vi "Main.vi"(8 "error in":errorcluster, 11 "TopUI in":refnum<class "TopUI.lvclass">) -> (0 "error out":errorcluster, 3 "TopUI out":refnum<class "TopUI.lvclass">)   [LabVIEW 2024, in "TopUI.lvclass"]
doc: "The <b>Queued Message Handler</b> of the Worker that owns this VI."
uses:
  TopUI.lvclass
  C:/Program Files (x86)/National Instruments/LabVIEW 2024/vi.lib/addons/_Workers/Library/Classes/Worker/Worker.lvclass
  TopUI.lvclass/TopUI.ctl
  Initialization Data.ctl
  Response Cases.ctl
  rql_NewAPIMHLCreate.ctl
  rql_UpdatePanelDisplay.ctl
  rql_ReadMeterValue.ctl
  rql_GetValueAvg.ctl
  <vilib>/addons/_Workers/Library/Classes/Message Queue/Message Queue.lvclass
  ooxxMeter/ooxxMeter.lvclass
  C:/Program Files (x86)/National Instruments/LabVIEW 2024/vi.lib/addons/_Workers/Library/Classes/Workers Object/Workers Object.lvclass
  C:/Users/chrismadlax/Desktop/LVSampleCode/Wokers50Demo/Workers/TopUI/TopUI.lvclass
panel:
  out "ValueAvg":dbl
  in  "GetValueAvg":bool
  out "MeterValue":dbl
  in  "ReadMeter":bool
  in  "Increment":bool
  out "Counter":dbl
  # "Public Request with respones"
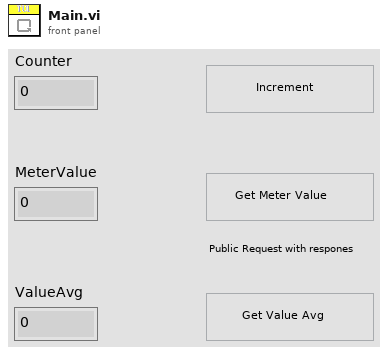
[diagram p1: front panel]
types:
  T1 = typedef "TopUI.lvclass/Initialization Data.ctl" = cluster{"Response Cases":T2}
  T2 = typedef "TopUI.lvclass/Response Cases.ctl" = cluster{"Placeholder - Can be deleted":string}
  T3 = typedef "TopUI.lvclass/rql_NewAPIMHLCreate.ctl" = cluster{"String":string}
  T4 = typedef "TopUI.lvclass/rql_UpdatePanelDisplay.ctl" = cluster{"String":string}
  T5 = typedef "TopUI.lvclass/rql_ReadMeterValue.ctl" = cluster{"String":string}
  T6 = typedef "TopUI.lvclass/rql_GetValueAvg.ctl" = cluster{"String":string}
  T7 = typedef "ooxxMeter.lvclass/rwr_ReadMeterValueNow Reply.ctl" = cluster{"String":string, "MeterValue":dbl}
  T8 = typedef "ooxxMeter.lvclass/rsp_ReturnValueAvg.ctl" = cluster{"String":string, "ValueAvg":dbl}
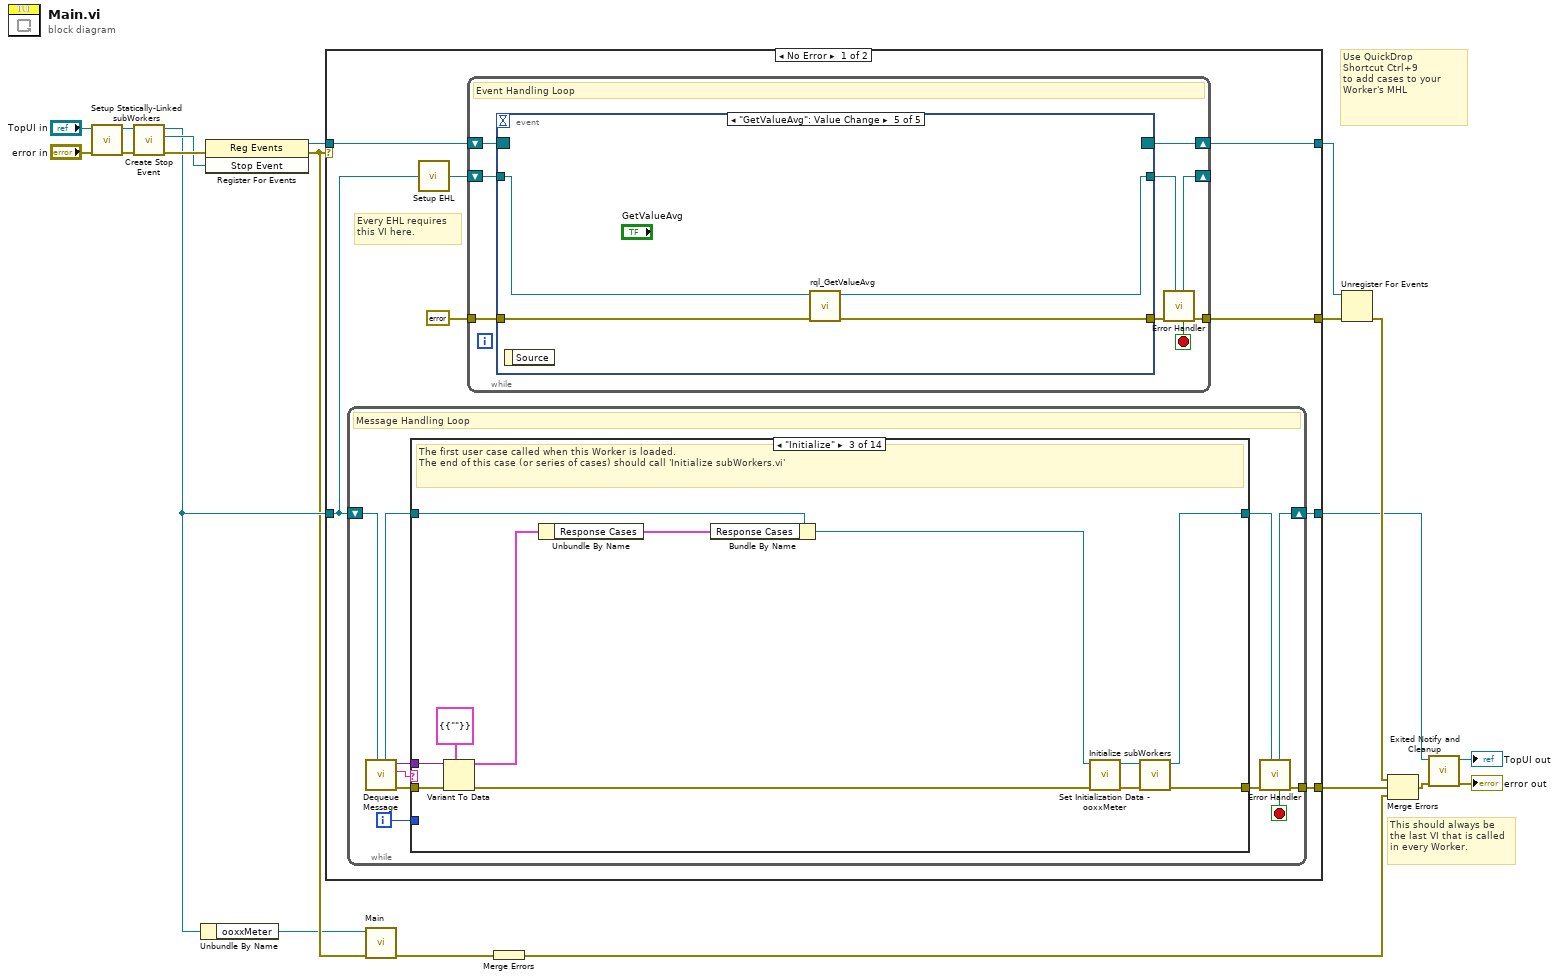
[diagram p0: block diagram]
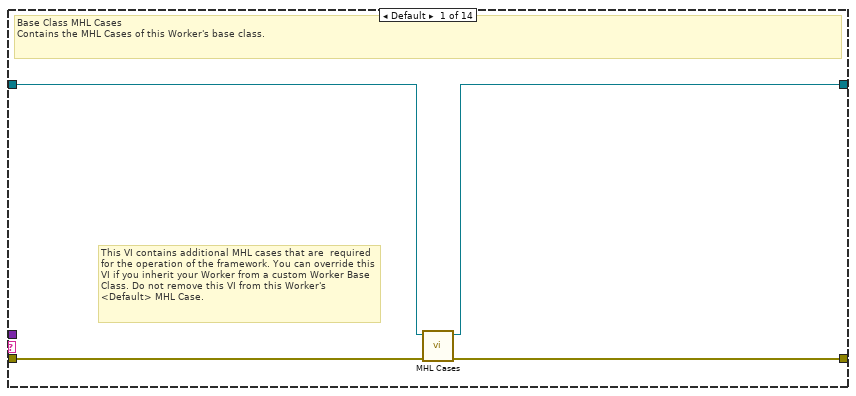
[diagram p2: hidden frame]
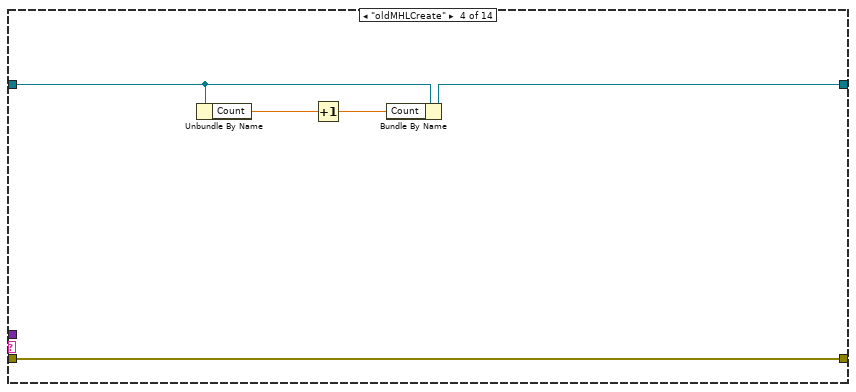
[diagram p4: hidden frame]
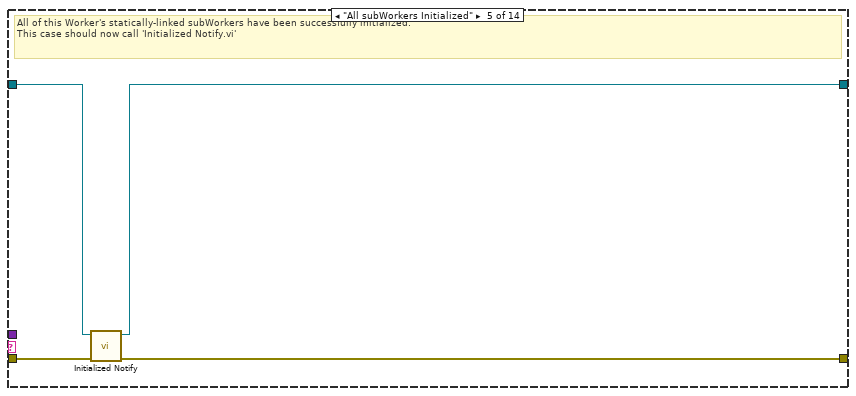
[diagram p5: hidden frame]
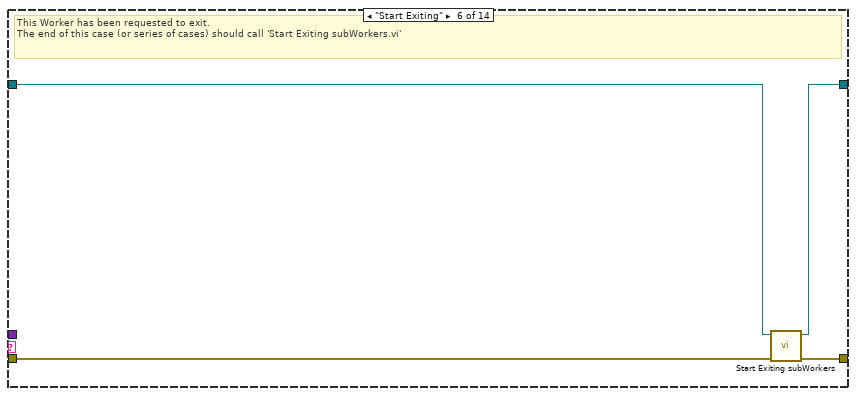
[diagram p6: hidden frame]
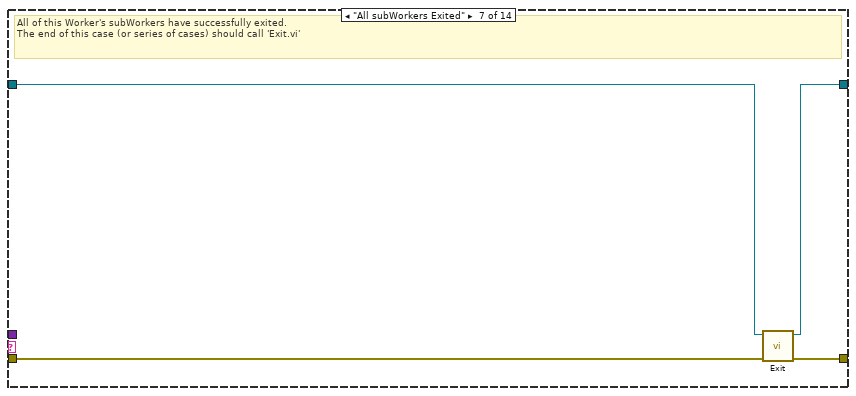
[diagram p7: hidden frame]
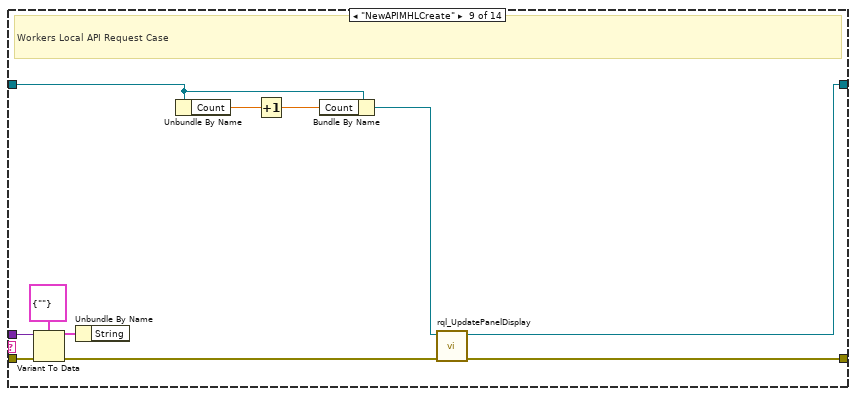
[diagram p9: hidden frame]
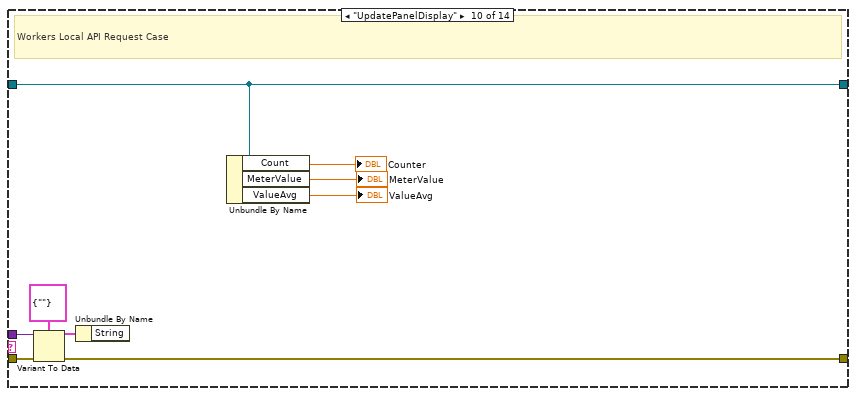
[diagram p10: hidden frame]
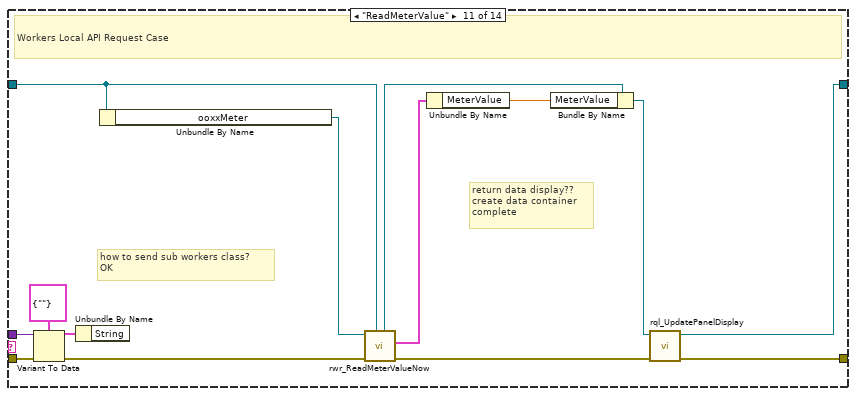
[diagram p11: hidden frame]
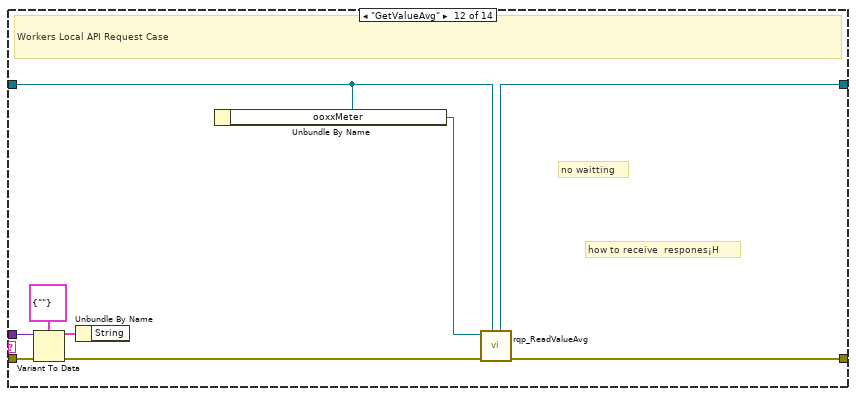
[diagram p12: hidden frame]
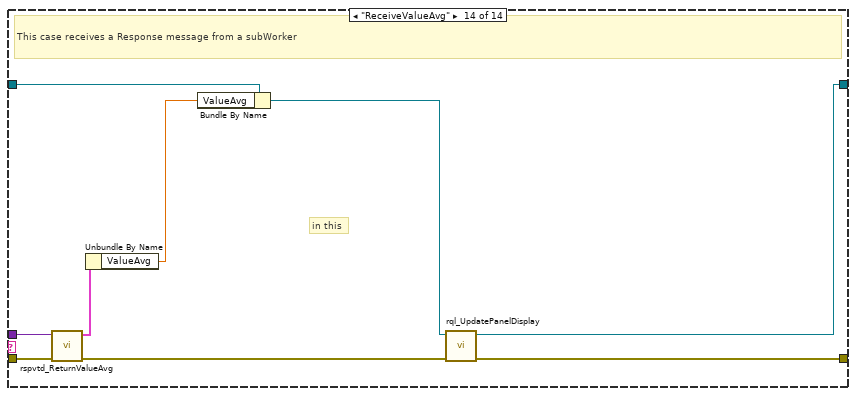
[diagram p14: hidden frame]
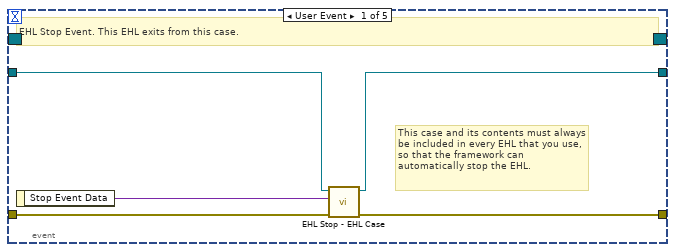
[diagram p15: hidden frame]
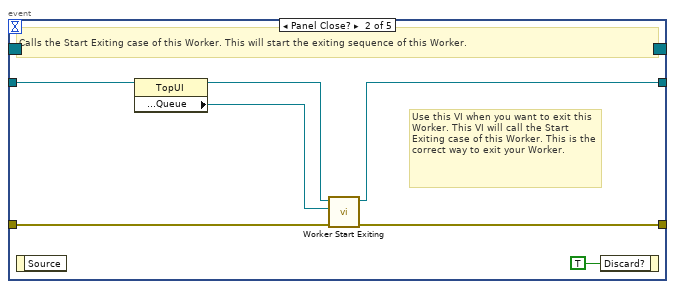
[diagram p16: hidden frame]
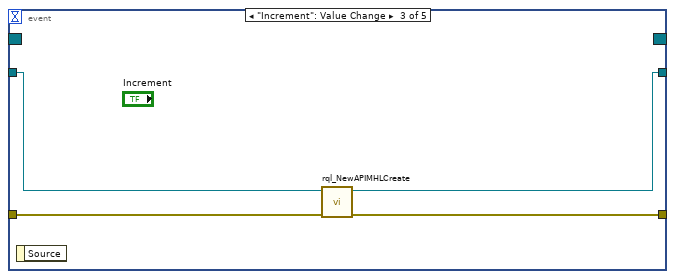
[diagram p17: hidden frame]
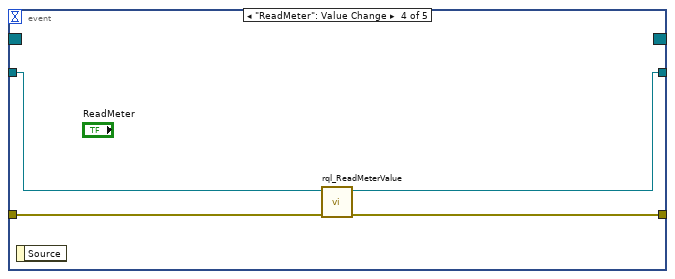
[diagram p18: hidden frame]
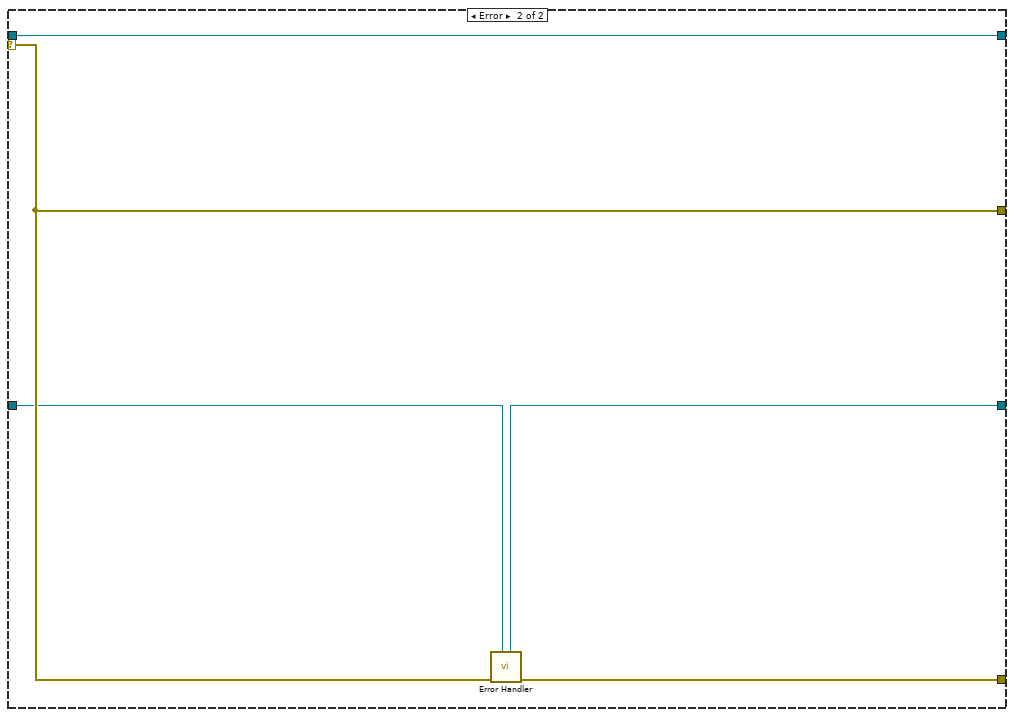
[diagram p19: hidden frame]
diagram:
  # "Use QuickDrop\nShortcut Ctrl+9\nto add cases to your\nWorker's MHL"
  # "This should always be the last VI that is called in every Worker."
  n1 = call "Setup Statically-Linked subWorkers.vi"("error in"="error in", "TopUI in"="TopUI in") -> ("error out"=w6:errorcluster, "TopUI out"=w4:refnum<class "TopUI.lvclass">)  [unwired: 8 in]
  n2 = call-dynamic "Create Stop Event.vi"("error in"=w6, "Worker"=w4) -> ("error out"=w15:errorcluster, "Stop Event"=w12:refnum<user-event>, "Worker out"=w9:refnum<class "TopUI.lvclass">)  [unwired: 7 in]
  n3 = Unbundle By Name(w9) -> ("ooxxMeter"=w1:refnum<class "ooxxMeter.lvclass">)
  n4 = register-events(error in=w15, w12) -> (reference out=w14:refnum<event-registration>, error out=w7:errorcluster)  [unwired: 1 in]
  n5 = case shown="No Error" w7 {
    tunnel: w9 -> [w23 w165]
    tunnel: [w21 w166] -> w13
    tunnel: w14 -> [w28 w167]
    tunnel: [w25 w168] -> w19
    tunnel: [w27 w167] -> w18
    tunnel: [w22 w164] -> w16
    selector: w7 -> [_ w168]
    frame No Error {
      # "Every EHL requires\nthis VI here."
      n6 = while {
        shift-right: [w37] -> w22
        shift-left: w23 -> [w39]
        tunnel: [w38] -> w21
        i -> [w30]
        stop <- w31 stop-if-true
        # "Message Handling Loop"
        n7 = call-dynamic "Dequeue Message.vi"("Worker"=w39) -> ("error out"=w36:errorcluster, "Case out"=w32:string, "Data out"=w29:variant, "Worker out"=w34:refnum<class "TopUI.lvclass">)  [unwired: 6 in, 1 out]
        n8 = case "Worker MHL Case Structure (DO NOT CHANGE LABEL NAME)" shown="\"Initialize\"" w32 {
          tunnel: w36 -> [w43 w44 w55 w62 w64 w67 w74 w76 w87 w96 w110 w119 w121 w130]
          tunnel: [w42 w44 w57 w62 w63 w70 w73 w76 w79 w95 w99 w114 w121 w124] -> w35
          tunnel: w34 -> [w41 w45 w54 w60 w66 w68 w72 w75 w82 w91 w103 w112 w120 w129]
          tunnel: [w40 w45 w56 w61 w65 w69 w71 w75 w77 w91 w97 w113 w120 w122] -> w33
          tunnel: w30 -> [_ _ _ _ _ _ _ _ _ _ _ _ _ _]
          tunnel: w29 -> [_ _ w52 _ _ _ _ _ w84 w93 w107 w116 _ w127]
          frame Default {
            # "This VI contains additional MHL cases that are  required for the operation of the framework. You can override this VI if you inherit your Worker from a custom Worker Base Class. Do not remove this VI from this Worker's <Default> MHL Case."
            # "Base Class MHL Cases\nContains the MHL Cases of this Worker's base class."
            n9 = call-dynamic "MHL Cases.vi"("error in"=w43, "Worker in"=w41) -> ("error out"=w42:errorcluster, "Worker out"=w40:refnum<class "TopUI.lvclass">)  [unwired: 8 in]
          }
          frame "------------ FRAMEWORK CASES -----------" {
            # "Start of Workers Framework Cases"
          }
          frame "Initialize" {
            # "The first user case called when this Worker is loaded.\nThe end of this case (or series of cases) should call 'Initialize subWorkers.vi'"
            n10 = Variant To Data(error in=w55, type=T1 {"Response Cases"={"Placeholder - Can be deleted"=""}} ("Initialization Data"), Variant=w52) -> (data=w51:T1, error out=w53:errorcluster)
            n11 = Unbundle By Name(w51) -> ("Response Cases"=w50:T2)
            n12 = Bundle By Name(cluster=w54, "Response Cases"=w50) -> (w46:refnum<class "TopUI.lvclass">)
            n13 = call "Set Initialization Data - ooxxMeter.vi"("error in"=w53, "TopUI in"=w46) -> ("error out"=w48:errorcluster, "TopUI out"=w47:refnum<class "TopUI.lvclass">)  [unwired: 8 in]
            n14 = call-dynamic "Initialize subWorkers.vi"("error in"=w48, "Worker"=w47) -> ("error out"=w57:errorcluster, "dup Worker out"=w56:refnum<class "TopUI.lvclass">)  [unwired: 8 in]
          }
          frame "oldMHLCreate" {
            n15 = Unbundle By Name(w60) -> ("Count"=w59:dbl)
            n16 = Increment(x=w59) -> (x+1=w58:dbl)
            n17 = Bundle By Name(cluster=w60, "Count"=w58) -> (w61:refnum<class "TopUI.lvclass">)
          }
          frame "All subWorkers Initialized" {
            # "All of this Worker's statically-linked subWorkers have been successfully initialized.\nThis case should now call 'Initialized Notify.vi'"
            n18 = call-dynamic "Initialized Notify.vi"("error in"=w64, "Worker"=w66) -> ("error out"=w63:errorcluster, "dup Worker out"=w65:refnum<class "TopUI.lvclass">)  [unwired: 8 in]
          }
          frame "Start Exiting" {
            # "This Worker has been requested to exit. \nThe end of this case (or series of cases) should call 'Start Exiting subWorkers.vi'"
            n19 = call-dynamic "Start Exiting subWorkers.vi"("error_in"=w67, "Worker"=w68) -> ("error out"=w70:errorcluster, "dup Worker out"=w69:refnum<class "TopUI.lvclass">)  [unwired: 8 in]
          }
          frame "All subWorkers Exited" {
            # "All of this Worker's subWorkers have successfully exited. \nThe end of this case (or series of cases) should call 'Exit.vi'"
            n20 = call-dynamic "Exit.vi"("error_in"=w74, "Worker"=w72) -> ("error out"=w73:errorcluster, "dup Worker out"=w71:refnum<class "TopUI.lvclass">)  [unwired: 8 in]
          }
          frame "------------- LOCAL API CASES -------------" {
            # "Start of Workers Local API Cases"
          }
          frame "NewAPIMHLCreate" {
            # "Workers Local API Request Case"
            n21 = Variant To Data(error in=w87, type=T3 {"String"=""} ("Data"), Variant=w84) -> (data=w83:T3, error out=w86:errorcluster)
            n22 = Unbundle By Name(w83) -> ()  [unwired: 1 out]
            n23 = Unbundle By Name(w82) -> ("Count"=w81:dbl)
            n24 = Increment(x=w81) -> (x+1=w80:dbl)
            n25 = Bundle By Name(cluster=w82, "Count"=w80) -> (w78:refnum<class "TopUI.lvclass">)
            n26 = call "rql_UpdatePanelDisplay.vi"("error in"=w86, "TopUI in"=w78) -> ("error out"=w79:errorcluster, "dup TopUI out"=w77:refnum<class "TopUI.lvclass">)  [unwired: 8 in]
          }
          frame "UpdatePanelDisplay" {
            # "Workers Local API Request Case"
            n27 = Variant To Data(error in=w96, type=T4 {"String"=""} ("Data"), Variant=w93) -> (data=w92:T4, error out=w95:errorcluster)
            n28 = Unbundle By Name(w92) -> ()  [unwired: 1 out]
            n29 = Unbundle By Name(w91) -> ("Count"=→"Counter":dbl, "MeterValue"=→"MeterValue":dbl, "ValueAvg"=→"ValueAvg":dbl)
          }
          frame "ReadMeterValue" {
            # "return data display??\ncreate data container\ncomplete"
            # "how to send sub workers class?\nOK"
            # "Workers Local API Request Case"
            n30 = Variant To Data(error in=w110, type=T5 {"String"=""} ("Data"), Variant=w107) -> (data=w106:T5, error out=w109:errorcluster)
            n31 = Unbundle By Name(w106) -> ()  [unwired: 1 out]
            n32 = Unbundle By Name(w103) -> ("ooxxMeter"=w102:refnum<class "ooxxMeter.lvclass">)
            n33 = call "rwr_ReadMeterValueNow.vi"("Caller in"=w103, "error in"=w109, "ooxxMeter in"=w102) -> ("error out"=w105:errorcluster, "Reply Data out"=w101:T7, "dup Caller out"=w104:refnum<class "TopUI.lvclass">)  [unwired: 5 in, 1 out]
            n34 = Unbundle By Name(w101) -> ("MeterValue"=w100:dbl)
            n35 = Bundle By Name(cluster=w104, "MeterValue"=w100) -> (w98:refnum<class "TopUI.lvclass">)
            n36 = call "rql_UpdatePanelDisplay.vi"("error in"=w105, "TopUI in"=w98) -> ("error out"=w99:errorcluster, "dup TopUI out"=w97:refnum<class "TopUI.lvclass">)  [unwired: 8 in]
          }
          frame "GetValueAvg" {
            # "how to receive  respones¡H"
            # "no waitting"
            # "Workers Local API Request Case"
            n37 = Variant To Data(error in=w119, type=T6 {"String"=""} ("Data"), Variant=w116) -> (data=w115:T6, error out=w118:errorcluster)
            n38 = Unbundle By Name(w115) -> ()  [unwired: 1 out]
            n39 = Unbundle By Name(w112) -> ("ooxxMeter"=w111:refnum<class "ooxxMeter.lvclass">)
            n40 = call "rqp_ReadValueAvg.vi"("Caller in"=w112, "error in"=w118, "ooxxMeter in"=w111) -> ("error out"=w114:errorcluster, "dup Caller out"=w113:refnum<class "TopUI.lvclass">)  [unwired: 6 in, 1 out]
          }
          frame "------------- RESPONSE CASES --------------" {
            # "Start of Workers Response Cases"
          }
          frame "ReceiveValueAvg" {
            # "in this"
            # "This case receives a Response message from a subWorker"
            n41 = call "rspvtd_ReturnValueAvg.vi"("error in"=w130, "Data in"=w127) -> ("error out"=w128:errorcluster, "Data out"=w126:T8)  [unwired: 8 in]
            n42 = Unbundle By Name(w126) -> ("ValueAvg"=w125:dbl)
            n43 = Bundle By Name(cluster=w129, "ValueAvg"=w125) -> (w123:refnum<class "TopUI.lvclass">)
            n44 = call "rql_UpdatePanelDisplay.vi"("error in"=w128, "TopUI in"=w123) -> ("error out"=w124:errorcluster, "dup TopUI out"=w122:refnum<class "TopUI.lvclass">)  [unwired: 8 in]
          }
        }
        n45 = call-dynamic "Error Handler.vi"("Worker"=w33, "error_in"=w35) -> ("error out"=w38:errorcluster, "Stop Loop"=w31:bool, "Worker out"=w37:refnum<class "TopUI.lvclass">)  [unwired: 7 in]
      }
      n46 = call-dynamic "Setup EHL.vi"("Worker"=w23) -> ("Worker out"=w24:refnum<class "TopUI.lvclass">)  [unwired: 14 in]
      n47 = while "Event Handling Loop" {
        shift-right: [w139] -> w27
        shift-left: w28 -> [w138]
        tunnel: [w134] -> w25
        tunnel: errorcluster {"status"=FALSE, "code"=0, "source"=""} ("error constant") -> [w136]
        shift-right: [w132] -> _
        shift-left: w24 -> [w137]
        stop <- w131 stop-if-true
        # "Event Handling Loop"
        n48 = event shown="[4] \"GetValueAvg\": Value Change" {
          selector: w138 -> [_ _ _ _ _]
          dyn-events: [_ _ _ _ _] -> w139
          timeout: _ -> [_ _ _ _ _]
          tunnel: [w143 w150 w154 w158 w162] -> w135
          tunnel: w136 -> [w144 w149 w155 w159 w163]
          tunnel: w137 -> [w142 w148 w153 w157 w161]
          tunnel: [w141 w147 w152 w156 w160] -> w133
          event User Event {
            # "This case and its contents must always be included in every EHL that you use, so that the framework can automatically stop the EHL."
            # "EHL Stop Event. This EHL exits from this case."
            n49 = event-data() -> ("Stop Event Data"=w140:variant)  [unwired: 1 in]
            n50 = call-dynamic "EHL Stop - EHL Case.vi"("error in"=w144, "Stop Event Data"=w140, "Worker"=w142) -> ("error out"=w143:errorcluster, "Worker out"=w141:refnum<class "TopUI.lvclass">)  [unwired: 7 in]
          }
          event Panel Close? {
            # "Use this VI when you want to exit this Worker. This VI will call the Start Exiting case of this Worker. This is the correct way to exit your Worker."
            # "Calls the Start Exiting case of this Worker. This will start the exiting sequence of this Worker."
            n51 = event-data() -> ()  [unwired: 1 in, 1 out]
            n52 = property class="TopUI"(reference=w148) -> (reference out=w146:refnum<class "TopUI.lvclass">, "Accessors:Read:Public API:Queue"=w145:refnum<class "Message Queue.lvclass">)  [unwired: 1 in, 1 out]
            n53 = call-dynamic "Worker Start Exiting.vi"("error_in"=w149, "Message Queue"=w145, "Worker"=w146) -> ("error out"=w150:errorcluster, "dup Worker out"=w147:refnum<class "TopUI.lvclass">)  [unwired: 7 in]
            n54 = event-data ("Event Filter Node")("Discard?"=TRUE) -> ()  [unwired: 1 in, 1 out]
          }
          event "Increment": Value Change {
            n55 = event-data() -> ()  [unwired: 1 in, 1 out]
            n56 = call "rql_NewAPIMHLCreate.vi"("error in"=w155, "TopUI in"=w153) -> ("error out"=w154:errorcluster, "dup TopUI out"=w152:refnum<class "TopUI.lvclass">)  [unwired: 8 in]
          }
          event "ReadMeter": Value Change {
            n57 = event-data() -> ()  [unwired: 1 in, 1 out]
            n58 = call "rql_ReadMeterValue.vi"("error in"=w159, "TopUI in"=w157) -> ("error out"=w158:errorcluster, "dup TopUI out"=w156:refnum<class "TopUI.lvclass">)  [unwired: 8 in]
          }
          event "GetValueAvg": Value Change {
            n59 = event-data() -> ()  [unwired: 1 in, 1 out]
            n60 = call "rql_GetValueAvg.vi"("error in"=w163, "TopUI in"=w161) -> ("error out"=w162:errorcluster, "dup TopUI out"=w160:refnum<class "TopUI.lvclass">)  [unwired: 8 in]
          }
        }
        n61 = call-dynamic "Error Handler.vi"("Worker"=w133, "error_in"=w135) -> ("error out"=w134:errorcluster, "Stop Loop"=w131:bool, "Worker out"=w132:refnum<class "TopUI.lvclass">)  [unwired: 7 in]
      }
    }
    frame Error {
      n62 = call-dynamic "Error Handler.vi"("Worker"=w165, "error_in"=w168) -> ("error out"=w166:errorcluster, "Worker out"=w164:refnum<class "TopUI.lvclass">)  [unwired: 7 in, 1 out]
    }
  }
  n63 = call-dynamic "Main.vi"("error in"=w7, "ooxxMeter in"=w1) -> ("error out"=w3:errorcluster)  [unwired: 8 in, 1 out]
  n64 = Merge Errors(w3) -> (w2:errorcluster)
  n65 = Unregister For Events(event registration refnum=w18, error in=w19) -> (error out=w20:errorcluster)
  n66 = Merge Errors(w20, w13, w2) -> (w17:errorcluster)
  n67 = call-dynamic "Exited Notify and Cleanup.vi"("error_in"=w17, "Worker"=w16) -> ("error out"=→"error out":errorcluster, "dup Worker out"=→"TopUI out":refnum<class "TopUI.lvclass">)  [unwired: 8 in]
